vi "ORS_GalvoPrepareScan_uw-1kp_Duo.vi"(0 "Galvo":T1={"x mirror"="Dev1/ao0", "y mirror"="Dev1/ao1", "trig out"="Dev1/port0/line2", "x mirror task"="", "y mirror task"="", "trig out task"="", "n_axis"=0, "params"={"n_lines"=500, "n_frames"=400, "force to zero"=FALSE, "Triggers_per_sweep"=1.0, "X center"=0.0, "X span"=3.4000000000000004, "Y center"=0.0, "Y span"=0.0, "flyb.lines"=40, "n_triggers"=1, "mode"=3, "offset"=0.0, "galvo phase"=0, "span factor"=0.0, "Custom trig."={"n_f to c. trig"=0, "c. trig length"=0, "c. trig interval"=0, "n_c. trig"=0}, "f_per_pos"=1, "n_dataset"=1, "flyback fr"=0}, "acq trig out"="Dev1/port0/line4", "acq trig out task"="", "sample array X"=[], "sample array Y"=[], "custom trig out"="", "custom trig out task"="", "FDML-box"="TCPIP0::10.153.218.51::23::SOCKET", "ACQ/Galvo"=enum."NI_DAQ", "acq trig out an task"="", "acq trig out an"="Dev1/ao2", "Galvo Trig input"="/Dev1/PFI1", "Galvo Clk input"="OnboardClock", "sample array Acq trig out an"=[]} {"params"."n_dataset" min=1; "params"."X center" format="%^_3g"; "params"."X span" format="%^_3g"; "params"."Y center" format="%^_3g"; "params"."Y span" format="%^_3g"}, 1 "SampQuant.SampMode":i32(ring)=10123 items=["Finite Samples"=10178, "Continuous Samples"=10123, "Hardware Timed Single Point"=12522], 3 "3D frame":i32=2, 5 "AO.DataXferMech":i32(ring)=12590 items=["DMA"=10054, "Interrupts"=10204, "Programmed I/O"=10264, "USB Bulk"=12590], 7 "Fast Axis/Slow Axis":bool, 9 "use_digi_trig":bool, 11 "error in":errorcluster, 13 "Trigger condition":i32=20) -> (4 "Galvo out":T1={"x mirror"="Dev1/ao0", "y mirror"="Dev1/ao1", "trig out"="Dev1/port0/line2", "x mirror task"="", "y mirror task"="", "trig out task"="", "n_axis"=0, "params"={"n_lines"=500, "n_frames"=400, "force to zero"=FALSE, "Triggers_per_sweep"=1.0, "X center"=0.0, "X span"=3.4000000000000004, "Y center"=0.0, "Y span"=0.0, "flyb.lines"=40, "n_triggers"=1, "mode"=3, "offset"=0.0, "galvo phase"=0, "span factor"=0.0, "Custom trig."={"n_f to c. trig"=0, "c. trig length"=0, "c. trig interval"=0, "n_c. trig"=0}, "f_per_pos"=1, "n_dataset"=1, "flyback fr"=0}, "acq trig out"="Dev1/port0/line4", "acq trig out task"="", "sample array X"=[], "sample array Y"=[], "custom trig out"="", "custom trig out task"="", "FDML-box"="TCPIP0::10.153.218.51::23::SOCKET", "ACQ/Galvo"=enum."NI_DAQ", "acq trig out an task"="", "acq trig out an"="Dev1/ao2", "Galvo Trig input"="/Dev1/PFI1", "Galvo Clk input"="OnboardClock", "sample array Acq trig out an"=[]} {"params"."n_dataset" min=1; "params"."X center" format="%^_3g"; "params"."X span" format="%^_3g"; "params"."Y center" format="%^_3g"; "params"."Y span" format="%^_3g"}, 6 "Galvo wfm":dbl[][](graph), 14 "Trigger Out":u32[][](graph), 15 "error out":errorcluster)   [LabVIEW 2021]
uses:
  Typedefs/ORS_Galvo.ctl
  Typedefs/ORS_Galvo_params.ctl
  <vilib>/Utility/error.llb/DialogType.ctl
  <vilib>/DAQmx/write.llb/DAQmx Write (Digital Bool 1Line 1Point).vi
  <vilib>/DAQmx/write.llb/DAQmx Write (Analog DBL 1Chan 1Samp).vi
  <vilib>/DAQmx/write.llb/DAQmx Write (Analog 2D DBL NChan NSamp).vi
  <vilib>/DAQmx/write.llb/DAQmx Write (Analog 1D DBL NChan 1Samp).vi
  <vilib>/DAQmx/write.llb/DAQmx Write (Digital 2D U32 NChan NSamp).vi
  <vilib>/DAQmx/write.llb/DAQmx Write (Analog 1D DBL 1Chan NSamp).vi
  <vilib>/DAQmx/miscellaneous.llb/DAQmx Fill In Error Info.vi
  <resource>/objmgr/daqmx.rc
panel:
  out "# samples":i32
  in  "SampQuant.SampMode 2":i32(ring)=10123 items=["Finite Samples"=10178, "Continuous Samples"=10123, "Hardware Timed Single Point"=12522]
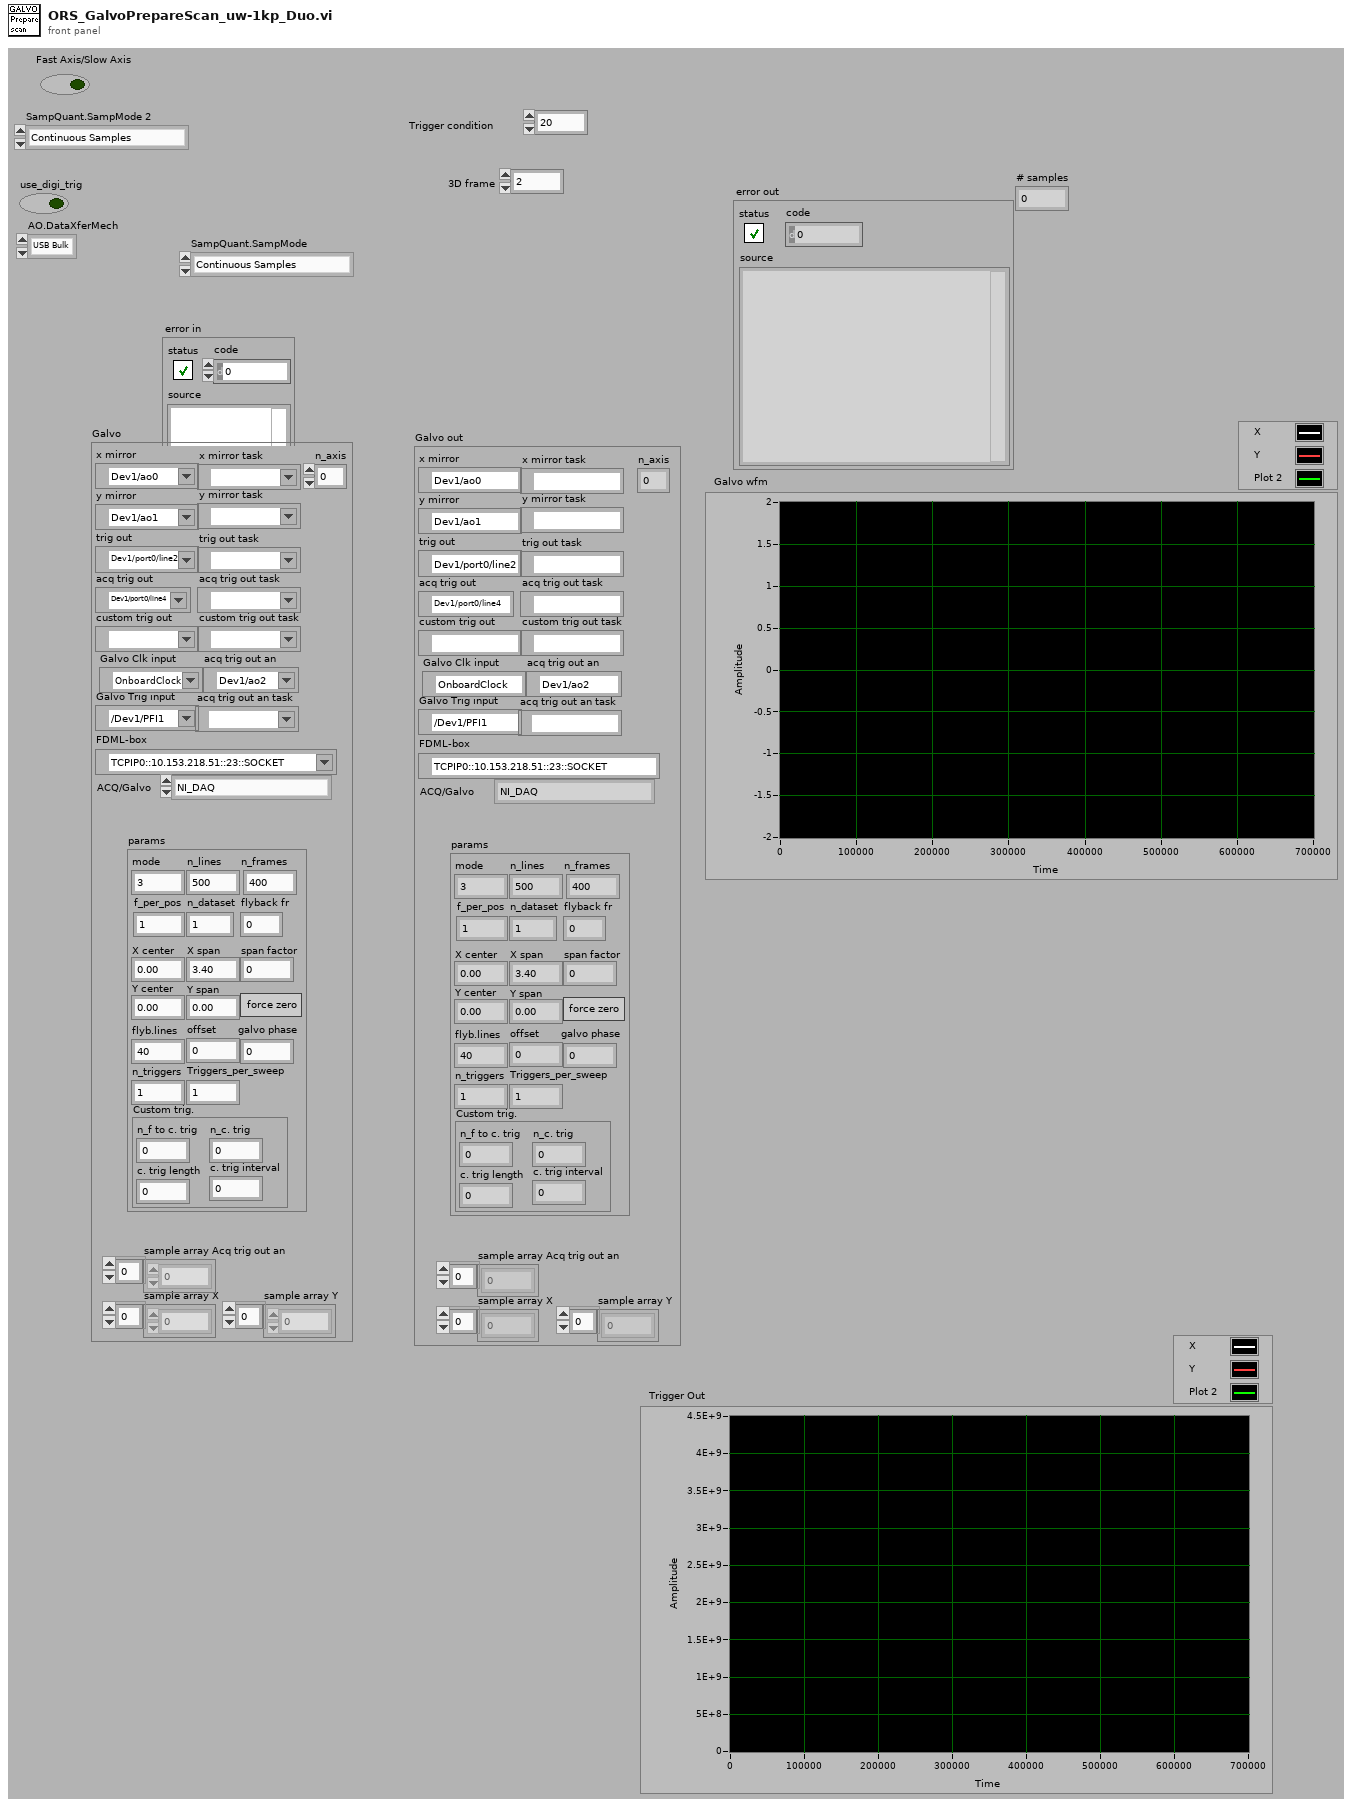
[diagram p1: front panel]
types:
  T1 = typedef "ORS_Galvo.ctl" = cluster{"x mirror":tag, "y mirror":tag, "trig out":tag, "x mirror task":refnum<k21>, "y mirror task":refnum<k21>, "trig out task":refnum<k21>, "n_axis":i32, "params":T2, "acq trig out":tag, "acq trig out task":refnum<k21>, "sample array X":dbl[], "sample array Y":dbl[], "custom trig out":tag, "custom trig out task":refnum<k21>, "FDML-box":refnum<visa-resource-name>, "ACQ/Galvo":enum16{"ADC/FDML", "NI_DAQ", "ADC"}, "acq trig out an task":refnum<k21>, "acq trig out an":tag, "Galvo Trig input":tag, "Galvo Clk input":tag, "sample array Acq trig out an":dbl[]}
  T2 = typedef "ORS_Galvo_params.ctl" = cluster{"n_lines":i32, "n_frames":i32, "force to zero":bool, "Triggers_per_sweep":dbl, "X center":dbl, "X span":dbl, "Y center":dbl, "Y span":dbl, "flyb.lines":i32, "n_triggers":i32, "mode":i32, "offset":dbl, "galvo phase":i32, "span factor":dbl, "Custom trig.":cluster{"n_f to c. trig":i32, "c. trig length":i32, "c. trig interval":i32, "n_c. trig":i32}, "f_per_pos":i32, "n_dataset":u32, "flyback fr":u16}
  T3 = typedef "DialogType.ctl" = u16
  T4 = cluster{"n_f to c. trig":i32, "c. trig length":i32, "c. trig interval":i32, "n_c. trig":i32}
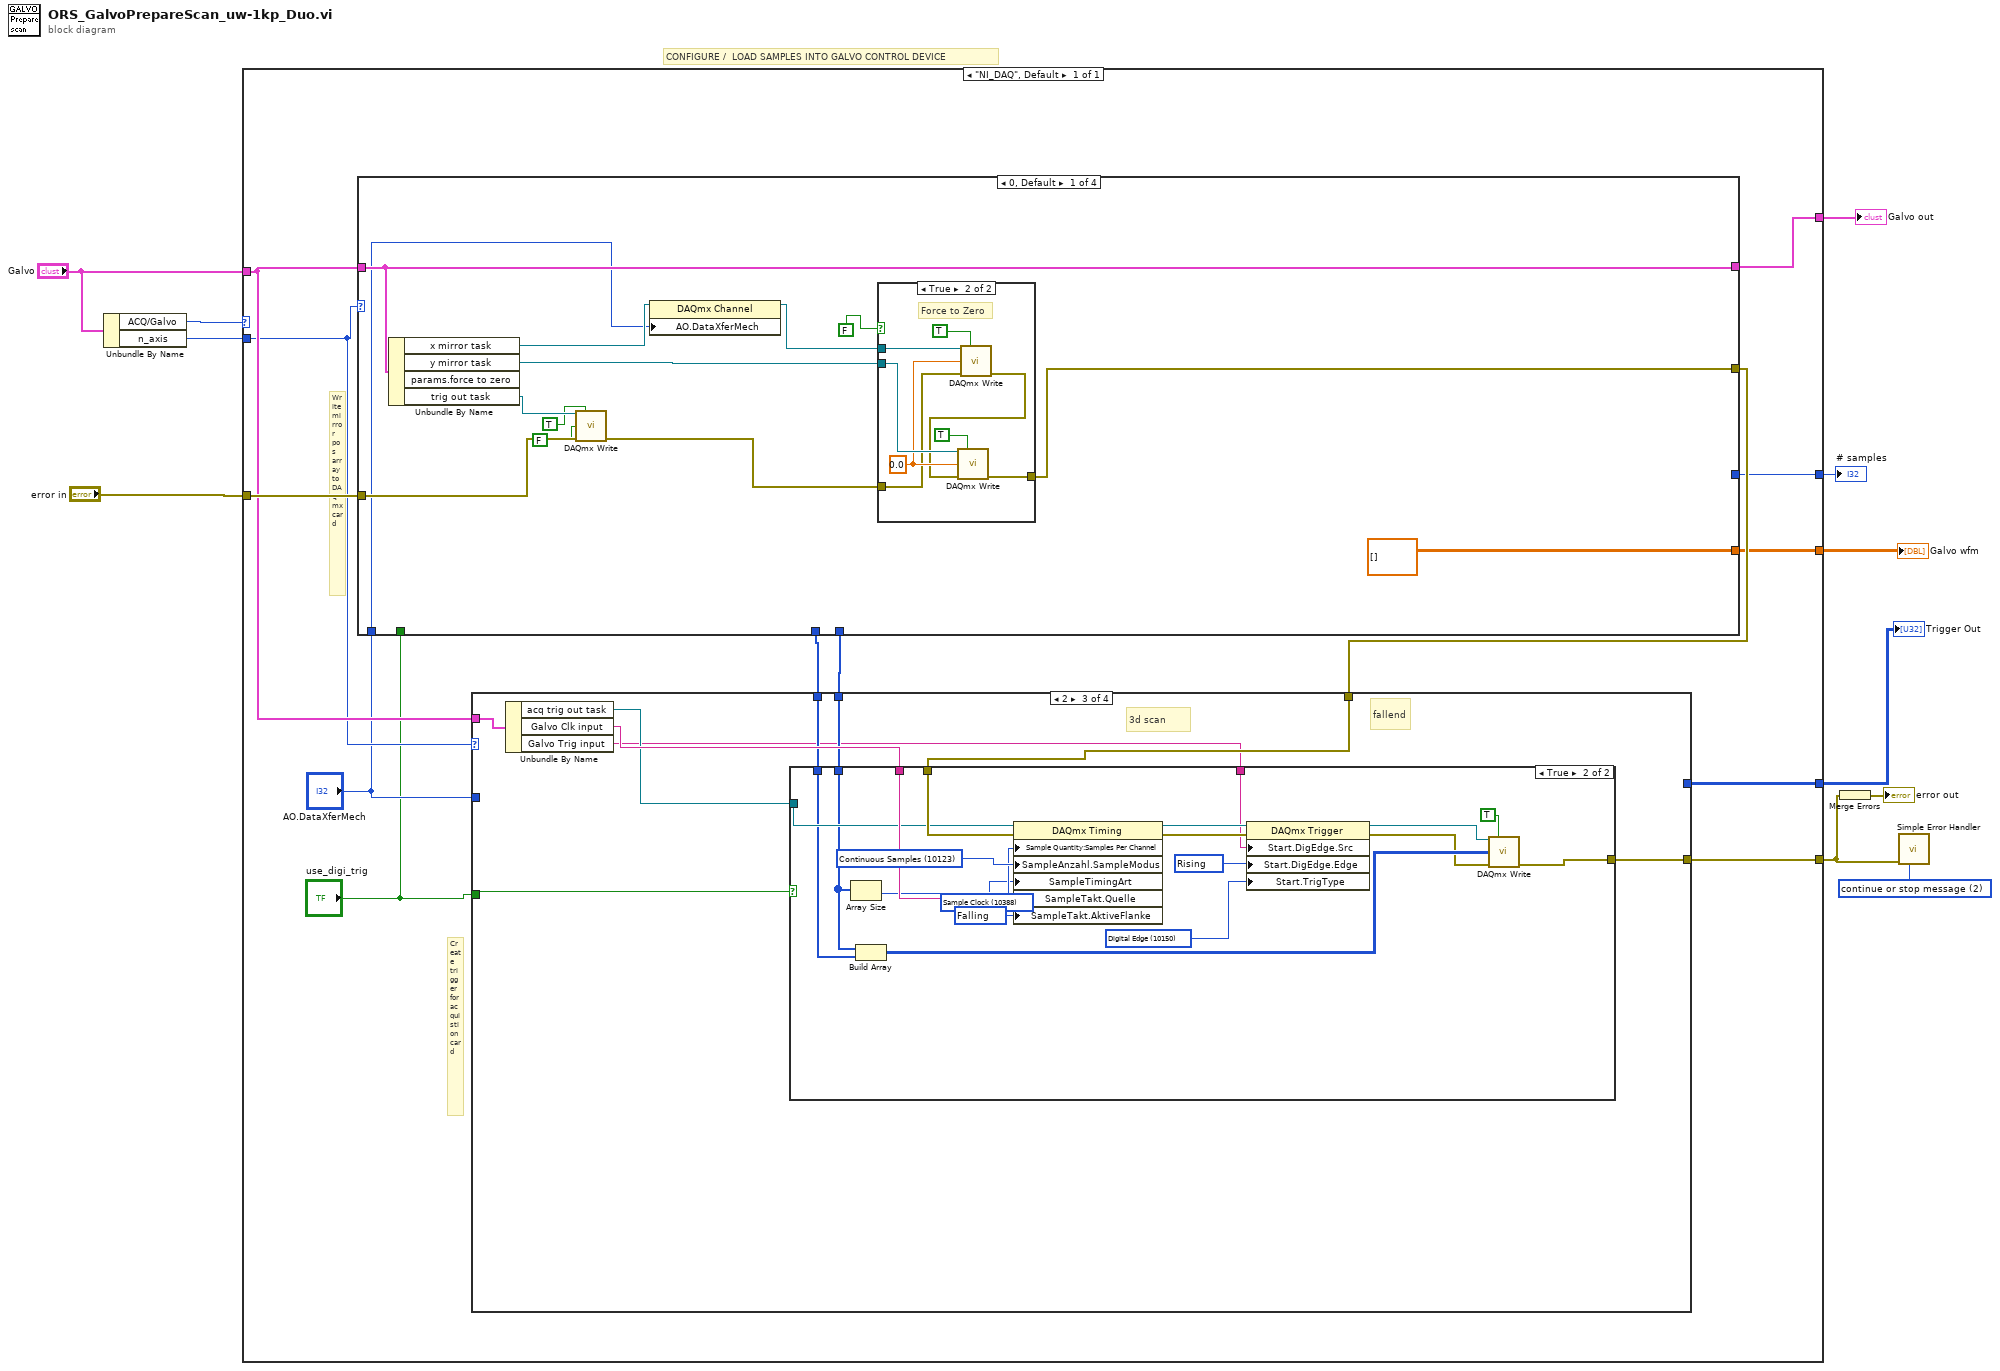
[diagram p0: block diagram]
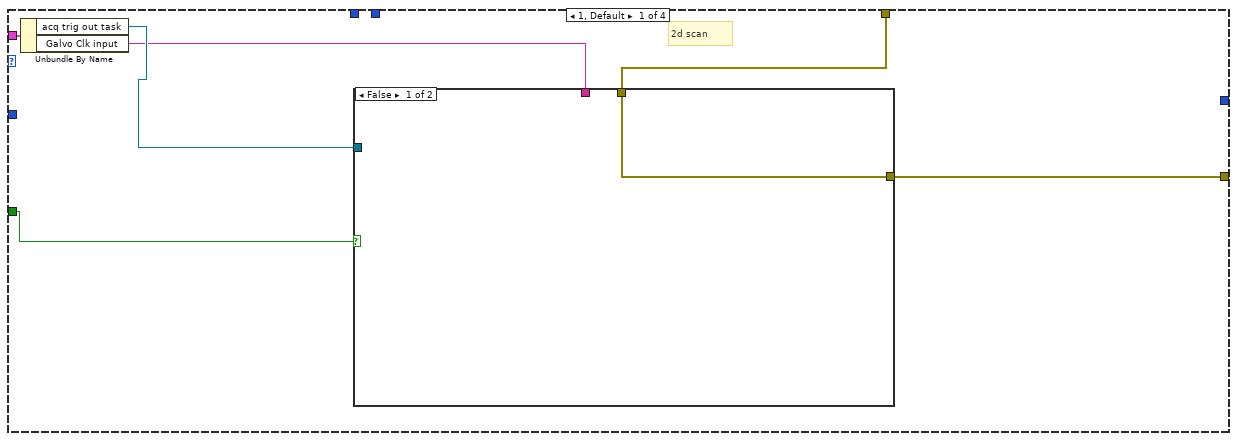
[diagram p2: hidden frame]
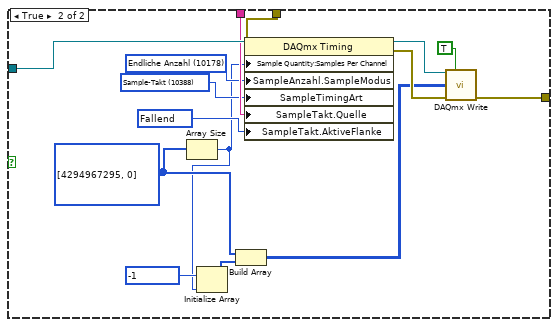
[diagram p3: hidden frame]
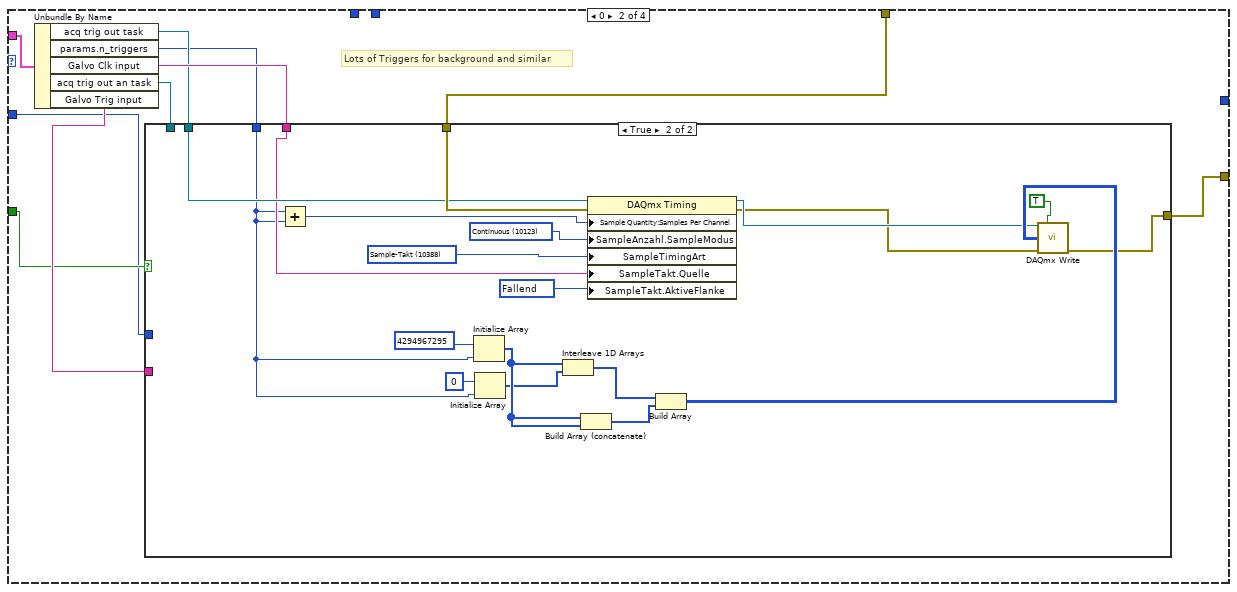
[diagram p4: hidden frame]
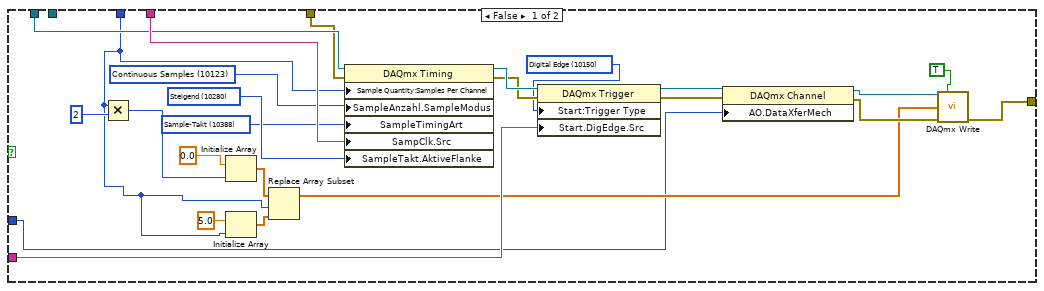
[diagram p5: hidden frame]
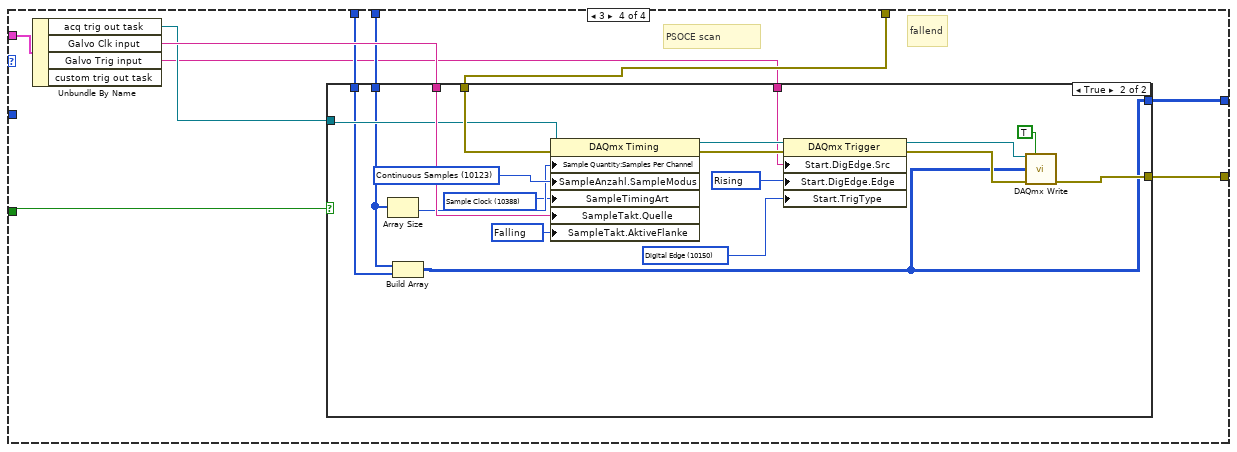
[diagram p7: hidden frame]
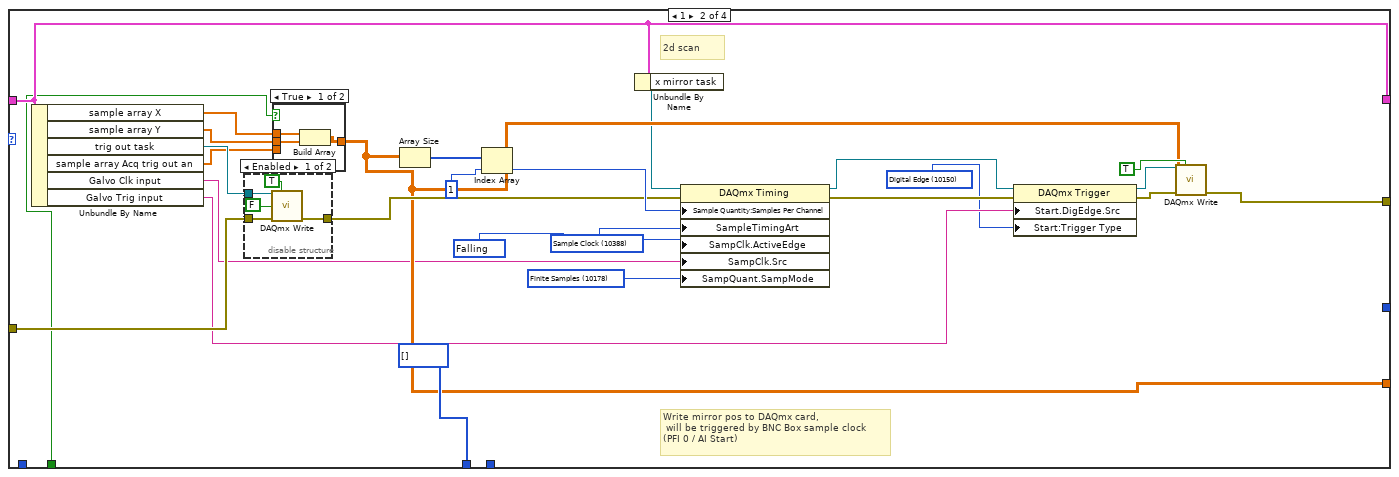
[diagram p10: hidden frame]
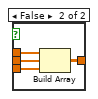
[diagram p12: hidden frame]
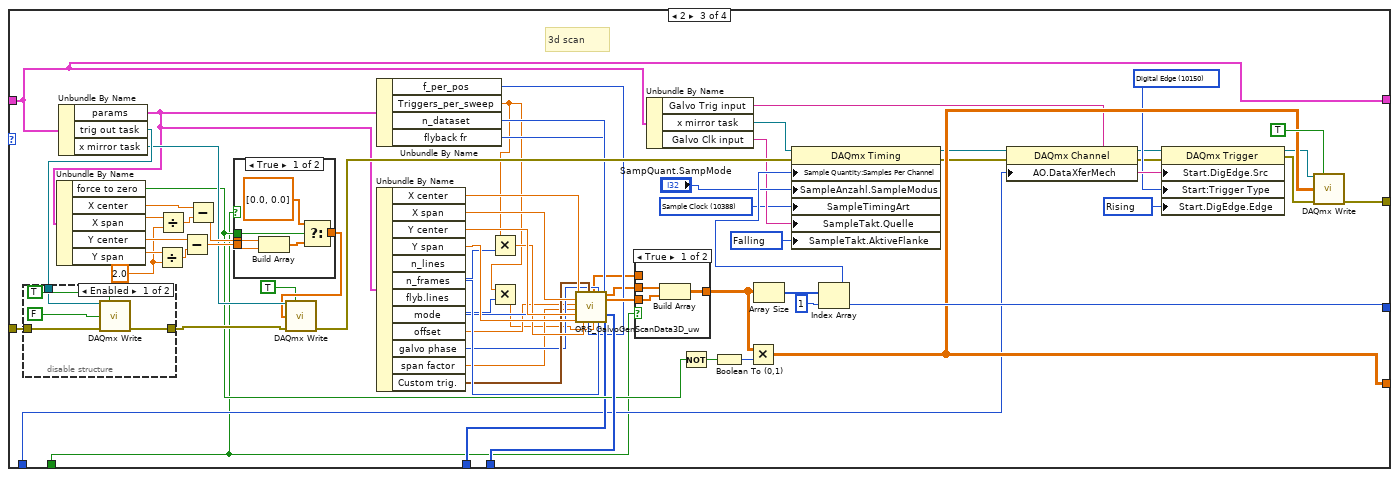
[diagram p13: hidden frame]
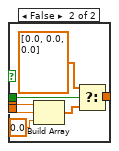
[diagram p15: hidden frame]
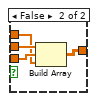
[diagram p16: hidden frame]
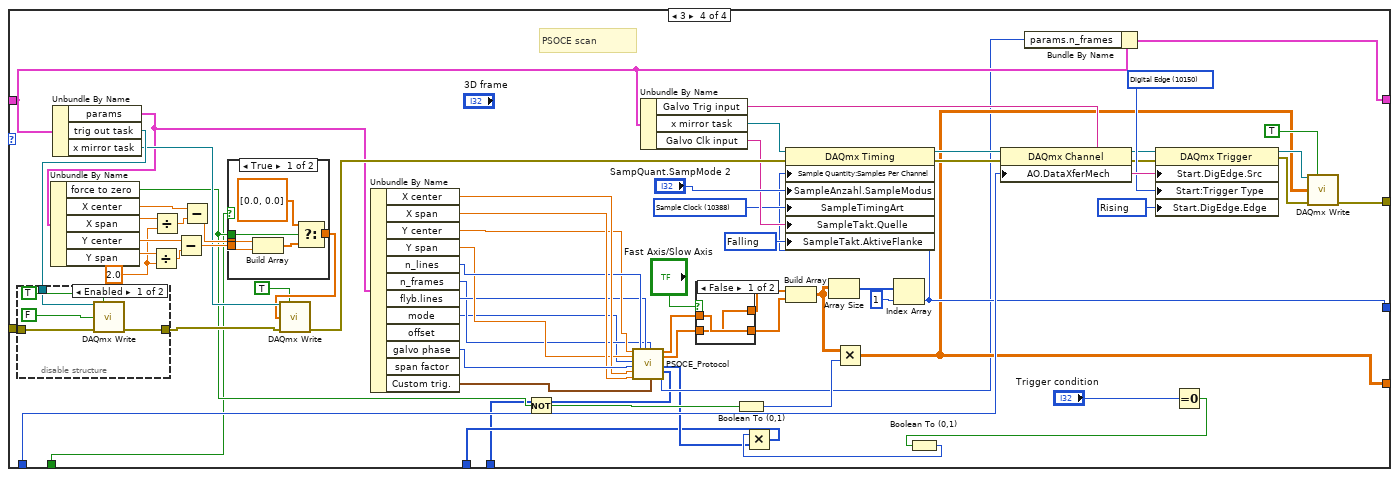
[diagram p17: hidden frame]
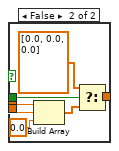
[diagram p20: hidden frame]
diagram:
  w8 = T3 2 items=["no dialog", "OK message", "continue or stop message", "OK message + warnings", "continue/stop + warnings"] ("type of dialog (OK msg:1)")
  # "CONFIGURE /  LOAD SAMPLES INTO GALVO CONTROL DEVICE"
  n1 = Unbundle By Name("Galvo") -> ("ACQ/Galvo"=w4:enum16{"ADC/FDML", "NI_DAQ", "ADC"}, "n_axis"=w3:i32)
  n2 = case shown="\"NI_DAQ\", Default" w4 {
    tunnel: "error in" -> [w24]
    tunnel: [w22] -> w9
    tunnel: [w19] -> w7
    tunnel: "Galvo" -> [w18]
    tunnel: [w17] -> w1
    tunnel: [w16] -> w6
    tunnel: w3 -> [w15]
    tunnel: [w12] -> w2
    frame "NI_DAQ", Default {
      # "Write mirror pos array to DAQmx card"
      # "Create trigger for acquistion card"
      n3 = case shown="0, Default" w15 {
        tunnel: w24 -> [w168 w206 w275 w344]
        tunnel: [w171 w204 w284 w339] -> w23
        tunnel: [w172 w193 w282 w328] -> w19
        tunnel: w18 -> [w172 w193 w282 w329]
        tunnel: [_ _ w276 w320] -> w21
        tunnel: [_ u32[] [] ("custom trig out") w253 w321] -> w20
        tunnel: [_ _ w244 w341] -> w17
        tunnel: [dbl[][] [] w195 w238 w340] -> w16
        tunnel: "AO.DataXferMech" -> [w160 _ w224 w343]
        tunnel: "use_digi_trig" -> [_ w182 w223 w342]
        frame 0, Default {
          n4 = Unbundle By Name(w172) -> ("x mirror task"=w164:refnum<k21>, "y mirror task"=w170:refnum<k21>, "trig out task"=w169:refnum<k21>)  [unwired: 1 out]
          n5 = call-poly <vilib>:"DAQmx Write.vi"("task/channels in"=w169, "auto start"=TRUE, "data"=FALSE, "error in"=w168) -> ("error out"=w167:errorcluster)  [unwired: 9 in, 2 out]
          n6 = property class="DAQmx Channel"(reference=w164, "AO.DataXferMech"=w160) -> (reference out=w163:refnum<k21>)  [unwired: 1 in, 1 out]
          n7 = case shown="True" FALSE {
            tunnel: w170 -> [_ w181]
            tunnel: w167 -> [w173 w175]
            tunnel: [w173 w179] -> w171
            tunnel: w163 -> [_ w177]
            frame False {
            }
            frame True {
              w176 = 0.0 ("t")
              # "Force to Zero"
              n8 = call-poly <vilib>:"DAQmx Write.vi"("task/channels in"=w177, "auto start"=TRUE, "data"=w176, "error in"=w175) -> ("error out"=w174:errorcluster)  [unwired: 9 in, 2 out]
              n9 = call-poly <vilib>:"DAQmx Write.vi"("task/channels in"=w181, "auto start"=TRUE, "data"=w176, "error in"=w174) -> ("error out"=w179:errorcluster)  [unwired: 9 in, 2 out]
            }
          }
        }
        frame 1 {
          w183 = 10150 items=["Analog Edge"=10099, "Digital Edge"=10150, "Digital Pattern"=10398, "Analog Window"=10103, "None"=10230] ("Start.TrigType")
          w190 = 10178 items=["Finite Samples"=10178, "Continuous Samples"=10123, "Hardware Timed Single Point"=12522] ("SampQuant.SampMode")
          w191 = 10388 items=["Sample Clock"=10388, "Burst Handshake"=12548, "Handshake"=10389, "Implicit"=10451, "On Demand"=10390, "Change Detection"=12504, "Pipelined Sample Clock"=14668] ("SampTimingType")
          w196 = 10171 items=["Rising"=10280, "Falling"=10171] ("SampClk.ActiveEdge")
          # "2d scan"
          # "Write mirror pos to DAQmx card,\n will be triggered by BNC Box sample clock\n(PFI 0 / AI Start)"
          n10 = Unbundle By Name(w193) -> ("sample array X"=w203:dbl[], "sample array Y"=w202:dbl[], "trig out task"=w207:refnum<k21>, "sample array Acq trig out an"=w194:dbl[], "Galvo Clk input"=w185:tag, "Galvo Trig input"=w186:tag)
          n11 = disable-structure shown="Enabled" {
            disable-tunnel: w207 -> [w212 _]
            disable-tunnel: w206 -> [w210 w213]
            disable-tunnel: [w208 w213] -> w198
            frame Enabled {
              n12 = call-poly <vilib>:"DAQmx Write.vi"("task/channels in"=w212, "auto start"=TRUE, "data"=FALSE, "error in"=w210) -> ("error out"=w208:errorcluster)  [unwired: 9 in, 2 out]
            }
            frame Disabled {
            }
          }
          n13 = case shown="True" w182 {
            tunnel: w203 -> [w216 w220]
            tunnel: w202 -> [w215 w219]
            tunnel: [w214 w218] -> w195
            tunnel: w194 -> [_ w217]
            frame True {
              n14 = Build Array(w216, w215) -> (w214:dbl[][])
            }
            frame False {
              n15 = Build Array(w220, w219, w217) -> (w218:dbl[][])
            }
          }
          n16 = Array Size(array=w195) -> (size(s)=w201:i32[])
          n17 = Index Array(array=w201, index=1) -> (element=w199:i32)
          n18 = Unbundle By Name(w193) -> ("x mirror task"=w192:refnum<k21>)
          n19 = property class="DAQmx Timing"(reference=w192, error in=w198, "Sample Quantity:Samples Per Channel"=w199, "SampleTimingArt"=w191, "SampClk.ActiveEdge"=w196, "SampClk.Src"=w185, "SampQuant.SampMode"=w190) -> (reference out=w184:refnum<k21>, error out=w188:errorcluster)
          n20 = property class="DAQmx Trigger"(reference=w184, error in=w188, "Start.DigEdge.Src"=w186, "Start:Trigger Type"=w183) -> (reference out=w189:refnum<k21>, error out=w187:errorcluster)
          n21 = call-poly <vilib>:"DAQmx Write.vi"("task/channels in"=w189, "auto start"=TRUE, "data"=w195, "error in"=w187) -> ("error out"=w204:errorcluster)  [unwired: 9 in, 2 out]
        }
        frame 2 {
          w221 = 10171 items=["Rising"=10280, "Falling"=10171] ("SampClk.ActiveEdge")
          w222 = 10388 items=["Sample Clock"=10388, "Burst Handshake"=12548, "Handshake"=10389, "Implicit"=10451, "On Demand"=10390, "Change Detection"=12504, "Pipelined Sample Clock"=14668] ("SampTimingType")
          w225 = 10280 items=["Rising"=10280, "Falling"=10171] ("Start.DigEdge.Edge")
          w231 = 10150 items=["Analog Edge"=10099, "Digital Edge"=10150, "Digital Pattern"=10398, "Analog Window"=10103, "None"=10230] ("Start.TrigType")
          w262 = 2.0
          # "3d scan"
          n22 = Unbundle By Name(w282) -> ("params"=w256:T2, "trig out task"=w274:refnum<k21>, "x mirror task"=w267:refnum<k21>)
          n23 = disable-structure shown="Enabled" {
            disable-tunnel: w275 -> [w290 w293]
            disable-tunnel: w274 -> [w289 _]
            disable-tunnel: [w288 w293] -> w273
            frame Enabled {
              n24 = call-poly <vilib>:"DAQmx Write.vi"("task/channels in"=w289, "auto start"=TRUE, "data"=FALSE, "error in"=w290) -> ("error out"=w288:errorcluster)  [unwired: 9 in, 2 out]
            }
            frame Disabled {
            }
          }
          n25 = Unbundle By Name(w256) -> ("force to zero"=w257:bool, "X center"=w271:dbl, "X span"=w263:dbl, "Y center"=w270:dbl, "Y span"=w266:dbl)
          n26 = Divide(x=w266, y=w262) -> (x/y=w265:dbl)
          n27 = Divide(x=w263, y=w262) -> (x/y=w264:dbl)
          n28 = Subtract(x=w270, y=w265) -> (x-y=w268:dbl)
          n29 = Subtract(x=w271, y=w264) -> (x-y=w269:dbl)
          n30 = case shown="True" w223 {
            tunnel: w269 -> [w299 w306]
            tunnel: w268 -> [w298 w305]
            tunnel: [w296 w303] -> w261
            tunnel: w257 -> [w295 w302]
            frame True {
              n31 = Build Array(w299, w298) -> (w297:dbl[])
              n32 = Select(t=dbl[] [0.0, 0.0] ("s? t:f"), s=w295, f=w297) -> (s? t:f=w296:dbl[])
            }
            frame False {
              n33 = Build Array(w306, w305, 0.0 ("element")) -> (w304:dbl[])
              n34 = Select(t=dbl[] [0.0, 0.0, 0.0] ("s? t:f"), s=w302, f=w304) -> (s? t:f=w303:dbl[])
            }
          }
          n35 = call-poly <vilib>:"DAQmx Write.vi"("task/channels in"=w267, "auto start"=TRUE, "data"=w261, "error in"=w273) -> ("error out"=w272:errorcluster)  [unwired: 9 in, 2 out]
          n36 = Unbundle By Name(w256) -> ("f_per_pos"=w247:i32, "Triggers_per_sweep"=w242:dbl, "n_dataset"=w246:u32, "flyback fr"=w245:u16)
          n37 = Unbundle By Name(w256) -> ("X center"=w281:dbl, "X span"=w280:dbl, "Y center"=w279:dbl, "Y span"=w278:dbl, "n_lines"=w255:i32, "n_frames"=w277:i32, "flyb.lines"=w241:i32, "mode"=w251:i32, "offset"=w248:dbl, "galvo phase"=w250:i32, "span factor"=w249:dbl, "Custom trig."=w252:T4)
          n38 = Multiply(x=w242, y=w255) -> (x*y=w254:dbl)
          n39 = Multiply(x=w242, y=w241) -> (x*y=w240:dbl)
          n40 = call "ORS_GalvoGenScanData3D_uw.vi"("x_center"=w281, "x_span"=w280, "offset"=w248, "span-factor"=w249, "y_center"=w279, "y_span"=w278, "mode"=w251, "n_lines"=w254, "Custom trig."=w252, "n_frames same y pos"=w247, "flyback_lines"=w240, "galvo phase"=w250, "n_frames"=w277, "n_3D scans"=w246, "flyback frames"=w245) -> ("t_data"=w237:dbl[], "x_data"=w239:dbl[], "y_data"=w283:dbl[], "trigger out"=w276:u32[], "custom trig out"=w253:u32[])
          n41 = case shown="True" w223 {
            tunnel: w283 -> [w309 w313]
            tunnel: [w308 w312] -> w260
            tunnel: w239 -> [w307 w311]
            tunnel: w237 -> [_ w310]
            frame True {
              n42 = Build Array(w307, w309) -> (w308:dbl[][])
            }
            frame False {
              n43 = Build Array(w311, w313, w310) -> (w312:dbl[][])
            }
          }
          n44 = Unbundle By Name(w282) -> ("Galvo Trig input"=w234:tag, "x mirror task"=w285:refnum<k21>, "Galvo Clk input"=w232:tag)
          n45 = Not(x=w257) -> (.not. x?=w258:bool)
          n46 = Boolean To (0,1)(Boolean=w258) -> (0, 1=w259:i16)
          n47 = Multiply(x=w260, y=w259) -> (x*y=w238:dbl[][])
          n48 = Array Size(array=w260) -> (size(s)=w243:i32[])
          n49 = Index Array(array=w243, index=1 ("Index")) -> (element=w244:i32)
          n50 = property class="DAQmx Timing"(reference=w285, error in=w272, "Sample Quantity:Samples Per Channel"=w244, "SampleAnzahl.SampleModus"="SampQuant.SampMode", "SampleTimingArt"=w222, "SampleTakt.Quelle"=w232, "SampleTakt.AktiveFlanke"=w221) -> (reference out=w230:refnum<k21>, error out=w229:errorcluster)
          n51 = property class="DAQmx Channel"(reference=w230, error in=w229, "AO.DataXferMech"=w224) -> (reference out=w228:refnum<k21>, error out=w227:errorcluster)
          n52 = property class="DAQmx Trigger"(reference=w228, error in=w227, "Start.DigEdge.Src"=w234, "Start:Trigger Type"=w231, "Start.DigEdge.Edge"=w225) -> (reference out=w236:refnum<k21>, error out=w235:errorcluster)
          n53 = call-poly <vilib>:"DAQmx Write.vi"("task/channels in"=w236, "auto start"=TRUE, "data"=w238, "error in"=w235) -> ("error out"=w284:errorcluster)  [unwired: 9 in, 2 out]
        }
        frame 3 {
          w345 = 10171 items=["Rising"=10280, "Falling"=10171] ("SampClk.ActiveEdge")
          w346 = 10388 items=["Sample Clock"=10388, "Burst Handshake"=12548, "Handshake"=10389, "Implicit"=10451, "On Demand"=10390, "Change Detection"=12504, "Pipelined Sample Clock"=14668] ("SampTimingType")
          w347 = 10280 items=["Rising"=10280, "Falling"=10171] ("Start.DigEdge.Edge")
          w353 = 10150 items=["Analog Edge"=10099, "Digital Edge"=10150, "Digital Pattern"=10398, "Analog Window"=10103, "None"=10230] ("Start.TrigType")
          w365 = 2.0
          # "PSOCE scan"
          n54 = Unbundle By Name(w329) -> ("params"=w360:T2, "trig out task"=w377:refnum<k21>, "x mirror task"=w370:refnum<k21>)
          n55 = disable-structure shown="Enabled" {
            disable-tunnel: w344 -> [w387 w390]
            disable-tunnel: w377 -> [w386 _]
            disable-tunnel: [w385 w390] -> w376
            frame Enabled {
              n56 = call-poly <vilib>:"DAQmx Write.vi"("task/channels in"=w386, "auto start"=TRUE, "data"=FALSE, "error in"=w387) -> ("error out"=w385:errorcluster)  [unwired: 9 in, 2 out]
            }
            frame Disabled {
            }
          }
          n57 = Unbundle By Name(w360) -> ("force to zero"=w361:bool, "X center"=w374:dbl, "X span"=w366:dbl, "Y center"=w373:dbl, "Y span"=w369:dbl)
          n58 = Divide(x=w369, y=w365) -> (x/y=w368:dbl)
          n59 = Divide(x=w366, y=w365) -> (x/y=w367:dbl)
          n60 = Subtract(x=w373, y=w368) -> (x-y=w371:dbl)
          n61 = Subtract(x=w374, y=w367) -> (x-y=w372:dbl)
          n62 = case shown="True" w342 {
            tunnel: w372 -> [w396 w403]
            tunnel: w371 -> [w395 w402]
            tunnel: [w393 w400] -> w364
            tunnel: w361 -> [w392 w399]
            frame True {
              n63 = Build Array(w396, w395) -> (w394:dbl[])
              n64 = Select(t=dbl[] [0.0, 0.0] ("s? t:f"), s=w392, f=w394) -> (s? t:f=w393:dbl[])
            }
            frame False {
              n65 = Build Array(w403, w402, 0.0 ("element")) -> (w401:dbl[])
              n66 = Select(t=dbl[] [0.0, 0.0, 0.0] ("s? t:f"), s=w399, f=w401) -> (s? t:f=w400:dbl[])
            }
          }
          n67 = call-poly <vilib>:"DAQmx Write.vi"("task/channels in"=w370, "auto start"=TRUE, "data"=w364, "error in"=w376) -> ("error out"=w375:errorcluster)  [unwired: 9 in, 2 out]
          n68 = Unbundle By Name(w360) -> ("X center"=w335:dbl, "X span"=w334:dbl, "Y center"=w332:dbl, "Y span"=w331:dbl, "n_lines"=w333:i32, "n_frames"=w326:i32, "flyb.lines"=w330:i32, "mode"=w314:i32, "galvo phase"=w336:i32, "Custom trig."=w337:T4)  [unwired: 2 out]
          n69 = Not(x=w361) -> (.not. x?=w362:bool)
          n70 = call "PSOCE_Protocol.vi"("y_center"=w332, "y_span"=w331, "mode"=w314, "galvo phase"=w336, "x_center"=w335, "x_span"=w334, "n_lines"=w333, "flyback_lines"=w330, "n frames"=w326, "Custom trig."=w337) -> ("x_data"=w317:dbl[], "y_data"=w316:dbl[], "trigger out"=w322:u32[], "custom trig out"=w320:u32[], "Overall Frames"=w327:i32)  [unwired: 5 in]
          n71 = Unbundle By Name(w329) -> ("Galvo Trig input"=w356:tag, "x mirror task"=w378:refnum<k21>, "Galvo Clk input"=w354:tag)
          n72 = case shown="False" "Fast Axis/Slow Axis" {
            tunnel: [w381 w384] -> w318
            tunnel: w317 -> [w382 w384]
            tunnel: w316 -> [w381 w383]
            tunnel: [w382 w383] -> w315
            frame False {
            }
            frame True {
            }
          }
          n73 = Boolean To (0,1)(Boolean=w362) -> (0, 1=w363:i16)
          n74 = Build Array(w318, w315) -> (w338:dbl[][])
          n75 = Array Size(array=w338) -> (size(s)=w359:i32[])
          n76 = Multiply(x=w338, y=w363) -> (x*y=w340:dbl[][])
          n77 = Index Array(array=w359, index=1 ("Index")) -> (element=w341:i32)
          n78 = property class="DAQmx Timing"(reference=w378, error in=w375, "Sample Quantity:Samples Per Channel"=w341, "SampleAnzahl.SampleModus"="SampQuant.SampMode 2", "SampleTimingArt"=w346, "SampleTakt.Quelle"=w354, "SampleTakt.AktiveFlanke"=w345) -> (reference out=w352:refnum<k21>, error out=w351:errorcluster)
          n79 = property class="DAQmx Channel"(reference=w352, error in=w351, "AO.DataXferMech"=w343) -> (reference out=w350:refnum<k21>, error out=w349:errorcluster)
          n80 = Bundle By Name(cluster=w329, "params.n_frames"=w327) -> (w328:T1)
          n81 = property class="DAQmx Trigger"(reference=w350, error in=w349, "Start.DigEdge.Src"=w356, "Start:Trigger Type"=w353, "Start.DigEdge.Edge"=w347) -> (reference out=w358:refnum<k21>, error out=w357:errorcluster)
          n82 = Equal To 0?(x="Trigger condition") -> (x = 0?=w324:bool)
          n83 = Boolean To (0,1)(Boolean=w324) -> (0, 1=w323:i16)
          n84 = Multiply(x=w323, y=w322) -> (x*y=w321:u32[])
          n85 = call-poly <vilib>:"DAQmx Write.vi"("task/channels in"=w358, "auto start"=TRUE, "data"=w340, "error in"=w357) -> ("error out"=w339:errorcluster)  [unwired: 9 in, 2 out]
        }
      }
      n86 = case shown="2" w15 {
        tunnel: w18 -> [w30 w56 w109 w139]
        tunnel: [w26 w55 w106 w136] -> w22
        tunnel: w23 -> [w28 w51 w108 w138]
        tunnel: w21 -> [_ _ w103 w133]
        tunnel: w20 -> [_ _ w104 w134]
        tunnel: "use_digi_trig" -> [w25 w48 w102 w132]
        tunnel: "AO.DataXferMech" -> [_ w47 _ _]
        tunnel: [_ _ _ w130] -> w12
        frame 1, Default {
          # "2d scan"
          n87 = Unbundle By Name(w30) -> ("acq trig out task"=w29:refnum<k21>, "Galvo Clk input"=w27:tag)
          n88 = case shown="False" w25 {
            tunnel: w29 -> [_ w46]
            tunnel: w28 -> [w31 w45]
            tunnel: w27 -> [_ w44]
            tunnel: [w31 w43] -> w26
            frame False {
            }
            frame True {
              w36 = u32[] [4294967295, 0] ("data")
              w40 = 10171 items=["Steigend"=10280, "Fallend"=10171] ("SampleTakt.AktiveFlanke")
              w41 = 10178 items=["Endliche Anzahl"=10178, "kontinuierlich"=10123, "Einzelwert (HW-getaktet)"=12522] ("SampleAnzahl.SampleModus")
              w42 = 10388 items=["Sample-Takt"=10388, "Burst-Handshake"=12548, "Handshake"=10389, "implizit"=10451, "1 Sample"=10390, "Änderungserkennung"=12504, "Sample-Takt in Pipeline"=14668] ("SampleTimingArt")
              n89 = Array Size(array=w36) -> (size(s)=w33:i32)
              n90 = Initialize Array(-1 ("Waveform"), w33) -> (w32:i32[])
              n91 = Build Array(w36, w32) -> (w35:u32[][])
              n92 = property class="DAQmx Timing"(reference=w46, error in=w45, "Sample Quantity:Samples Per Channel"=w33, "SampleAnzahl.SampleModus"=w41, "SampleTimingArt"=w42, "SampleTakt.Quelle"=w44, "SampleTakt.AktiveFlanke"=w40) -> (reference out=w39:refnum<k21>, error out=w38:errorcluster)
              n93 = call-poly <vilib>:"DAQmx Write.vi"("task/channels in"=w39, "auto start"=TRUE, "data"=w35, "error in"=w38) -> ("error out"=w43:errorcluster)  [unwired: 9 in, 2 out]
            }
          }
        }
        frame 0 {
          # "Lots of Triggers for background and similar"
          n94 = Unbundle By Name(w56) -> ("acq trig out task"=w50:refnum<k21>, "params.n_triggers"=w49:i32, "Galvo Clk input"=w54:tag, "acq trig out an task"=w53:refnum<k21>, "Galvo Trig input"=w52:tag)
          n95 = case shown="True" w48 {
            tunnel: [w81 w86] -> w55
            tunnel: w54 -> [w80 w85]
            tunnel: w53 -> [w79 _]
            tunnel: w52 -> [w78 _]
            tunnel: w51 -> [w61 w88]
            tunnel: w50 -> [_ w87]
            tunnel: w49 -> [w58 w84]
            tunnel: w47 -> [w57 _]
            frame False {
              w62 = 10150 items=["Analog Edge"=10099, "Digital Edge"=10150, "Digital Pattern"=10398, "Analog Window"=10103, "None"=10230] ("Start.TrigType")
              w71 = 10123 items=["Finite Samples"=10178, "Continuous Samples"=10123, "Hardware Timed Single Point"=12522] ("SampQuant.SampMode")
              w75 = 10280 items=["Steigend"=10280, "Fallend"=10171] ("SampleTakt.AktiveFlanke")
              w74 = 10388 items=["Sample-Takt"=10388, "Burst-Handshake"=12548, "Handshake"=10389, "implizit"=10451, "1 Sample"=10390, "Änderungserkennung"=12504, "Sample-Takt in Pipeline"=14668] ("SampleTimingArt")
              n96 = Multiply(x=w58, y=2) -> (x*y=w59:i32)
              n97 = Initialize Array(0.0, w59) -> (w65:dbl[])
              n98 = Initialize Array(5.0, w58) -> (w64:dbl[])
              n99 = Replace Array Subset(array=w65, new element=w64, index=w58) -> (w63:dbl[])
              n100 = property class="DAQmx Timing"(reference=w79, error in=w61, "Sample Quantity:Samples Per Channel"=w58, "SampleAnzahl.SampleModus"=w71, "SampleTimingArt"=w74, "SampClk.Src"=w80, "SampleTakt.AktiveFlanke"=w75) -> (reference out=w73:refnum<k21>, error out=w72:errorcluster)
              n101 = property class="DAQmx Trigger"(reference=w73, error in=w72, "Start:Trigger Type"=w62, "Start.DigEdge.Src"=w78) -> (reference out=w70:refnum<k21>, error out=w69:errorcluster)
              n102 = property class="DAQmx Channel"(reference=w70, error in=w69, "AO.DataXferMech"=w57) -> (reference out=w68:refnum<k21>, error out=w67:errorcluster)
              n103 = call-poly <vilib>:"DAQmx Write.vi"("task/channels in"=w68, "auto start"=TRUE, "data"=w63, "error in"=w67) -> ("error out"=w81:errorcluster)  [unwired: 9 in, 2 out]
            }
            frame True {
              w91 = 10171 items=["Steigend"=10280, "Fallend"=10171] ("SampleTakt.AktiveFlanke")
              w90 = 10123 items=["Finite samplies"=10178, "Continuous"=10123, "Einzelwert (HW-getaktet)"=12522] ("SampleAnzahl.SampleModus")
              w89 = 10388 items=["Sample-Takt"=10388, "Burst-Handshake"=12548, "Handshake"=10389, "implizit"=10451, "1 Sample"=10390, "Änderungserkennung"=12504, "Sample-Takt in Pipeline"=14668] ("SampleTimingArt")
              n104 = Add(x=w84, y=w84) -> (x+y=w99:i32)
              n105 = Initialize Array(u32 4294967295 ("Waveform"), w84) -> (w100:u32[])
              n106 = Initialize Array(u32 0 ("Waveform"), w84) -> (w96:u32[])
              n107 = Interleave 1D Arrays(w100, w96) -> (w95:u32[])
              n108 = Build Array (concatenate)(w100, w100) -> (w97:u32[])
              n109 = property class="DAQmx Timing"(reference=w87, error in=w88, "Sample Quantity:Samples Per Channel"=w99, "SampleAnzahl.SampleModus"=w90, "SampleTimingArt"=w89, "SampleTakt.Quelle"=w85, "SampleTakt.AktiveFlanke"=w91) -> (reference out=w83:refnum<k21>, error out=w82:errorcluster)
              n110 = Build Array(w95, w97) -> (w98:u32[][])
              n111 = call-poly <vilib>:"DAQmx Write.vi"("task/channels in"=w83, "auto start"=TRUE, "data"=w98, "error in"=w82) -> ("error out"=w86:errorcluster)  [unwired: 9 in, 2 out]
            }
          }
        }
        frame 2 {
          # "fallend"
          # "3d scan"
          n112 = Unbundle By Name(w109) -> ("acq trig out task"=w105:refnum<k21>, "Galvo Clk input"=w107:tag, "Galvo Trig input"=w101:tag)
          n113 = case shown="True" w102 {
            tunnel: w108 -> [w110 w129]
            tunnel: w107 -> [_ w128]
            tunnel: [w110 w127] -> w106
            tunnel: w105 -> [_ w126]
            tunnel: w104 -> [_ w125]
            tunnel: w103 -> [_ w124]
            tunnel: w101 -> [_ w115]
            frame False {
            }
            frame True {
              w111 = 10171 items=["Rising"=10280, "Falling"=10171] ("SampClk.ActiveEdge")
              w112 = 10388 items=["Sample Clock"=10388, "Burst Handshake"=12548, "Handshake"=10389, "Implicit"=10451, "On Demand"=10390, "Change Detection"=12504, "Pipelined Sample Clock"=14668] ("SampTimingType")
              w123 = 10123 items=["Finite Samples"=10178, "Continuous Samples"=10123, "Hardware Timed Single Point"=12522] ("SampQuant.SampMode")
              w113 = 10150 items=["Analog Edge"=10099, "Digital Edge"=10150, "Digital Pattern"=10398, "Analog Window"=10103, "None"=10230] ("Start.TrigType")
              w114 = 10280 items=["Rising"=10280, "Falling"=10171] ("Start.DigEdge.Edge")
              n114 = Array Size(array=w124) -> (size(s)=w120:i32)
              n115 = Build Array(w124, w125) -> (w121:u32[][])
              n116 = property class="DAQmx Timing"(reference=w126, error in=w129, "Sample Quantity:Samples Per Channel"=w120, "SampleAnzahl.SampleModus"=w123, "SampleTimingArt"=w112, "SampleTakt.Quelle"=w128, "SampleTakt.AktiveFlanke"=w111) -> (reference out=w117:refnum<k21>, error out=w118:errorcluster)
              n117 = property class="DAQmx Trigger"(reference=w117, error in=w118, "Start.DigEdge.Src"=w115, "Start.DigEdge.Edge"=w114, "Start.TrigType"=w113) -> (reference out=w116:refnum<k21>, error out=w119:errorcluster)
              n118 = call-poly <vilib>:"DAQmx Write.vi"("task/channels in"=w116, "auto start"=TRUE, "data"=w121, "error in"=w119) -> ("error out"=w127:errorcluster)  [unwired: 9 in, 2 out]
            }
          }
        }
        frame 3 {
          # "fallend"
          # "PSOCE scan"
          n119 = Unbundle By Name(w139) -> ("acq trig out task"=w135:refnum<k21>, "Galvo Clk input"=w137:tag, "Galvo Trig input"=w131:tag)  [unwired: 1 out]
          n120 = case shown="True" w132 {
            tunnel: w138 -> [w140 w159]
            tunnel: w137 -> [_ w158]
            tunnel: [w140 w157] -> w136
            tunnel: w135 -> [_ w156]
            tunnel: w134 -> [_ w155]
            tunnel: w133 -> [_ w154]
            tunnel: w131 -> [_ w146]
            tunnel: [_ w141] -> w130
            frame False {
            }
            frame True {
              w142 = 10171 items=["Rising"=10280, "Falling"=10171] ("SampClk.ActiveEdge")
              w143 = 10388 items=["Sample Clock"=10388, "Burst Handshake"=12548, "Handshake"=10389, "Implicit"=10451, "On Demand"=10390, "Change Detection"=12504, "Pipelined Sample Clock"=14668] ("SampTimingType")
              w153 = 10123 items=["Finite Samples"=10178, "Continuous Samples"=10123, "Hardware Timed Single Point"=12522] ("SampQuant.SampMode")
              w144 = 10150 items=["Analog Edge"=10099, "Digital Edge"=10150, "Digital Pattern"=10398, "Analog Window"=10103, "None"=10230] ("Start.TrigType")
              w145 = 10280 items=["Rising"=10280, "Falling"=10171] ("Start.DigEdge.Edge")
              n121 = Array Size(array=w154) -> (size(s)=w151:i32)
              n122 = Build Array(w154, w155) -> (w141:u32[][])
              n123 = property class="DAQmx Timing"(reference=w156, error in=w159, "Sample Quantity:Samples Per Channel"=w151, "SampleAnzahl.SampleModus"=w153, "SampleTimingArt"=w143, "SampleTakt.Quelle"=w158, "SampleTakt.AktiveFlanke"=w142) -> (reference out=w148:refnum<k21>, error out=w149:errorcluster)
              n124 = property class="DAQmx Trigger"(reference=w148, error in=w149, "Start.DigEdge.Src"=w146, "Start.DigEdge.Edge"=w145, "Start.TrigType"=w144) -> (reference out=w147:refnum<k21>, error out=w150:errorcluster)
              n125 = call-poly <vilib>:"DAQmx Write.vi"("task/channels in"=w147, "auto start"=TRUE, "data"=w141, "error in"=w150) -> ("error out"=w157:errorcluster)  [unwired: 9 in, 2 out]
            }
          }
        }
      }
    }
  }
  "Galvo out" <- w7
  "Galvo wfm" <- w6
  "Trigger Out" <- w2
  "# samples" <- w1
  n126 = Merge Errors(w9) -> (→"error out":errorcluster)
  n127 = call <vilib>:"Simple Error Handler.vi"("type of dialog (OK msg:1)"=w8, "error in (no error)"=w9) -> ()  [unwired: 3 in, 5 out]
